vi "Set_All_List_Symbols.vi"(10 "symbol value":u16, 11 "MulticolumnListbox in":refnum<vi>) -> ()   [LabVIEW 2013]
doc: "Sets all the list symbols to value"
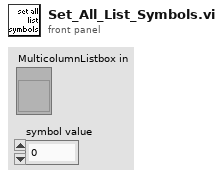
[diagram p1: front panel]
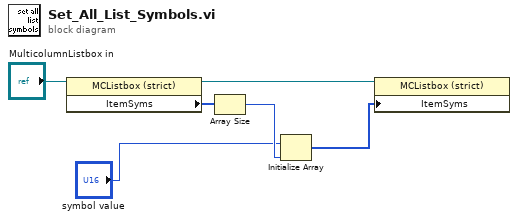
[diagram p0: block diagram]
diagram:
  n1 = property on="Property Node" class="MCListbox (strict)"(reference="MulticolumnListbox in") -> (reference out=w5:refnum<vi>, "ItemSyms"=w4:i32[])  [unwired: 1 in, 1 out]
  n2 = Array Size(array=w4) -> (size(s)=w3:i32)
  n3 = Initialize Array("symbol value", w3) -> (w1:u16[])
  n4 = property on="Property Node" class="MCListbox (strict)"(reference=w5, "ItemSyms"=w1) -> ()  [unwired: 1 in, 2 out]
